vi "mod_Create Mask for MSK Example.vi"(0 "Ramp Time  (sym)":dbl format="%.2f", 5 "Burst Length  (sym)":dbl format="%.2f", 9 "interpolation":T1(ring), 11 "dt":dbl format="%.2f") -> (4 "upper mask":dbl[](array[numeric]) format="%.2f", 6 "ideal":dbl[](array[numeric]) format="%.2f", 8 "lower mask":dbl[](array[numeric]) format="%.2f", 10 "ideal profile definition":cluster{"time":dbl, "power (dB)":dbl}[](array[cluster]) {"power (dB)" format="%.2f"; "time" format="%.2f"})   [LabVIEW 2020, in "niDMT.lvlib"]
uses:
  <vilib>/addons/Modulation/niDMT.lvlib
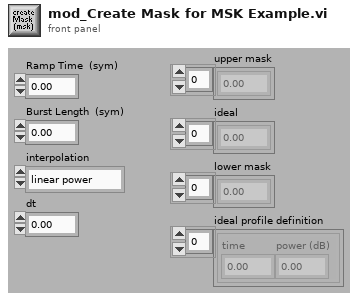
[diagram p1: front panel]
types:
  T1 = enum16{"linear power", "linear voltage", "linear dB"}
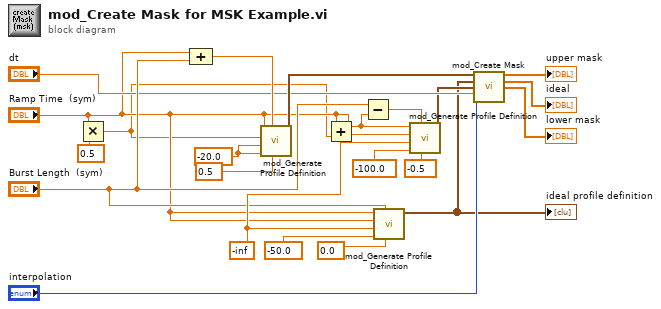
[diagram p0: block diagram]
diagram:
  w16 = -inf ("off level")
  w17 = -20.0 ("off level")
  n1 = Multiply(x="Ramp Time  (sym)", y=0.5) -> (x*y=w1:dbl)
  n2 = Compound Arithmetic op=ADD("Ramp Time  (sym)", "Burst Length  (sym)") -> (w14:dbl)
  n3 = call <vilib>:"mod_Generate Profile Definition.vi"("on level"=0.5, "burst length"=w14, "ramp start level"=w17, "off level"=w17, "off time"=w1, "ramp time"="Ramp Time  (sym)") -> ("profile definition"=w10:cluster{"time":dbl, "power (dB)":dbl}[])  [unwired: 5 out]
  n4 = Add(x="Ramp Time  (sym)", y=w1) -> (x+y=w4:dbl)
  n5 = Subtract(x="Burst Length  (sym)", y="Ramp Time  (sym)") -> (x-y=w15:dbl)
  n6 = call <vilib>:"mod_Generate Profile Definition.vi"("on level"=0.0, "burst length"="Burst Length  (sym)", "ramp start level"=-50.0, "off level"=w16, "off time"="Ramp Time  (sym)", "ramp time"="Ramp Time  (sym)") -> ("profile definition"=w5:cluster{"time":dbl, "power (dB)":dbl}[])  [unwired: 5 out]
  "ideal profile definition" <- w5
  n7 = call <vilib>:"mod_Generate Profile Definition.vi"("on level"=-0.5, "burst length"=w15, "ramp start level"=-100.0, "off level"=w16, "off time"=w4, "ramp time"="Ramp Time  (sym)") -> ("profile definition"=w6:cluster{"time":dbl, "power (dB)":dbl}[])  [unwired: 5 out]
  n8 = call <vilib>:"mod_Create Mask.vi"("upper mask definition"=w10, "ideal profile definition"=w5, "lower mask definition"=w6, "dt"="dt", "interpolation"="interpolation") -> ("upper mask"=→"upper mask":dbl[], "ideal"=→"ideal":dbl[], "lower mask"=→"lower mask":dbl[])  [unwired: 8 out]
